vi "Read Coils.vi"(7 "unit ID":u8, 8 "error in":errorcluster, 9 "number of inputs":u16, 10 "starting address":u16, 11 "Modbus master in":refnum<class "Modbus Master.lvclass">) -> (0 "error out":errorcluster, 2 "coils":bool[](array[boolean]), 3 "Modbus master out":refnum<class "Modbus Master.lvclass">)   [LabVIEW 2013, in "Modbus Library - Advance.lvlib" / "Modbus Master.lvclass"]
doc: "Reads <B>number of inputs</B> coils starting at <B>starting address</B> from the device."
uses:
  Modbus Master.lvclass
  Modbus Master.lvclass/Modbus Master.ctl
  Modbus API.lvclass/Modbus API.ctl
  Transmission Data Unit/Transmission Data Unit.lvclass/Transmission Data Unit.ctl
  Transmission Data Unit/Transmission Data Unit.lvclass
  Modbus API.lvclass
  Master Function Definition/Master Function Definition.lvclass
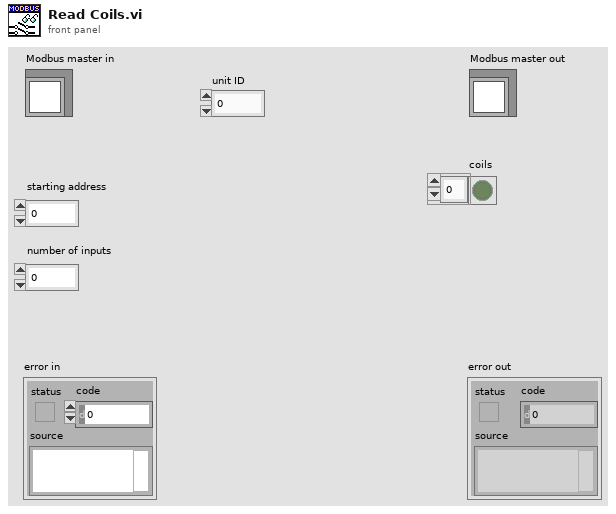
[diagram p1: front panel]
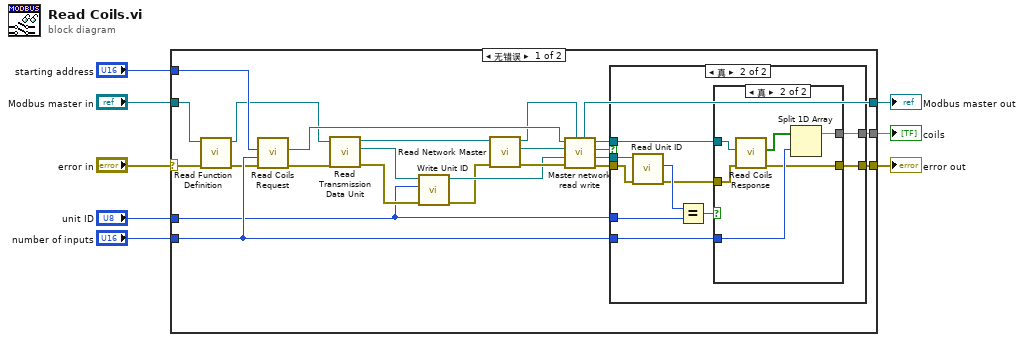
[diagram p0: block diagram]
diagram:
  n1 = case shown="无错误" "error in" {
    selector: "error in" -> [w25 w52]
    tunnel: [w24 w52] -> w6
    tunnel: [w22 w51] -> w7
    tunnel: "Modbus master in" -> [w26 w51]
    tunnel: "starting address" -> [w32 _]
    tunnel: "number of inputs" -> [w31 _]
    tunnel: [w30 _] -> w5
    tunnel: "unit ID" -> [w9 _]
    frame No Error {
      n2 = call "Read Function Definition.vi"("error in"=w25, "Modbus master in"=w26) -> ("error out"=w21:errorcluster, "Modbus master out"=w18:refnum<class "Modbus Master.lvclass">)  [unwired: 7 in, 1 out]
      n3 = call "Read Coils Request.vi"("error in"=w21, "Number of coils"=w31, "Starting Address"=w32) -> ("error out"=w16:errorcluster, "modbus data unit out"=w29:refnum<class "Modbus Data Unit.lvclass">)  [unwired: 7 in]
      n4 = call "Read Transmission Data Unit.vi"("error in"=w16, "Modbus instance in"=w18) -> ("error out"=w13:errorcluster, "transmission data unit"=w14:refnum<class "Transmission Data Unit.lvclass">, "Modbus instance out"=w19:refnum<class "Modbus Master.lvclass">)  [unwired: 7 in]
      n5 = call "Write Unit ID.vi"("error in"=w13, "unit ID"=w9, "transmission data unit in"=w14) -> ("error out"=w11:errorcluster, "transmission data unit out"=w12:refnum<class "Transmission Data Unit.lvclass">)  [unwired: 7 in]
      n6 = call "Read Network Master.vi"("error in"=w11, "Modbus master in"=w19) -> ("error out"=w20:errorcluster, "network master"=w23:refnum<class "Network Master.lvclass">, "Modbus master out"=w17:refnum<class "Modbus Master.lvclass">)  [unwired: 7 in]
      n7 = call "Master network read write.vi"("Modbus master in"=w17, "error in"=w20, "transmission data unit in"=w12, "network master in"=w23, "Modbus data unit in"=w29) -> ("error out"=w27:errorcluster, "transmission data unit out"=w10:refnum<class "Transmission Data Unit.lvclass">, "PDU Valid?"=w15:bool, "Modbus data unit out"=w28:refnum<class "Modbus Data Unit.lvclass">, "Modbus master out"=w22:refnum<class "Modbus Master.lvclass">)  [unwired: 2 in]
      n8 = case shown="真" w15 {
        tunnel: w31 -> [_ w43]
        tunnel: [_ w42] -> w30
        tunnel: w28 -> [_ w41]
        tunnel: w27 -> [w33 w38]
        tunnel: [w33 w40] -> w24
        tunnel: w10 -> [_ w39]
        tunnel: w9 -> [_ w37]
        frame False {
        }
        frame True {
          n9 = call "Read Unit ID.vi"("error in"=w38, "transmission data unit in"=w39) -> ("error out"=w34:errorcluster, "unit ID"=w36:u8)  [unwired: 7 in, 1 out]
          n10 = Equal?(x=w36, y=w37) -> (x = y?=w35:bool)
          n11 = case shown="真" w35 {
            tunnel: w43 -> [_ w50]
            tunnel: [_ w49] -> w42
            tunnel: w41 -> [_ w47]
            tunnel: [w44 w46] -> w40
            tunnel: w34 -> [w44 w45]
            frame False {
            }
            frame True {
              n12 = call "Read Coils Response.vi"("error in"=w45, "modbus data unit in"=w47) -> ("error out"=w46:errorcluster, "Data"=w48:bool[])  [unwired: 8 in]
              n13 = Split 1D Array(array=w48, index=w50) -> (first subarray=w49:bool[])  [unwired: 1 out]
            }
          }
        }
      }
    }
    frame Error {
    }
  }
  "error out" <- w6
  "Modbus master out" <- w7
  "coils" <- w5
